vi "Read Array.vi"(8 "error in (no error)":errorcluster, 11 "JSON Value In":refnum<class "JSON Value.lvclass">) -> (0 "error out":errorcluster, 2 "Array":refnum<class "JSON Value.lvclass">[](array[class]), 3 "JSON Value Out":refnum<class "JSON Value.lvclass">)   [LabVIEW 2011, in "JSON Value.lvclass"]
doc: "Returns the elements of a JSON array as an array of <b>JSON Values</b>\n\nCopyright 2012 James David Powell, Shaun Rumbell and Ton Plomp\nMore information on http://lavag.org/topic/16217-cr-json-labview"
uses:
  JSON Value.lvclass
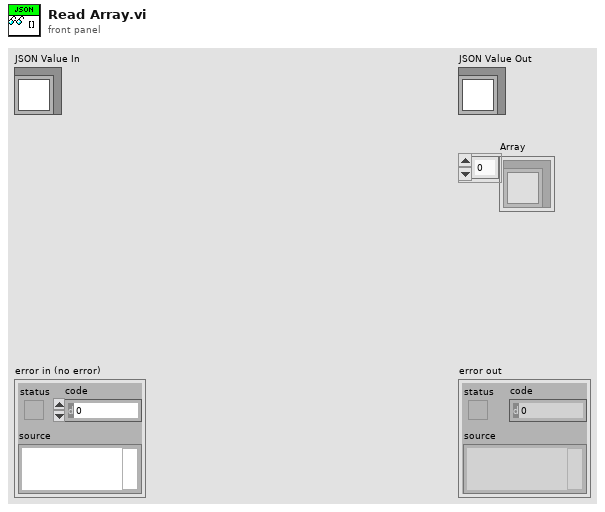
[diagram p1: front panel]
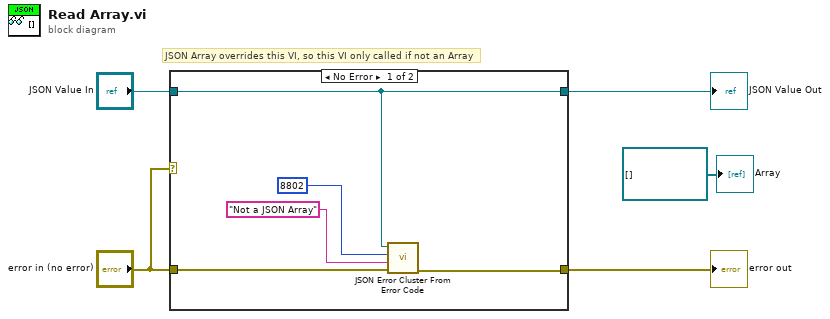
[diagram p0: block diagram]
diagram:
  # "JSON Array overrides this VI, so this VI only called if not an Array"
  n1 = case shown="No Error" "error in (no error)" {
    tunnel: "error in (no error)" -> [w8 w11]
    tunnel: [w7 w11] -> w5
    tunnel: "JSON Value In" -> [w6 w12]
    tunnel: [w6 w12] -> w3
    frame No Error {
      n2 = call "JSON Error Cluster From Error Code.vi"("error in (no error)"=w8, "Error message"="Not a JSON Array", "JSON error code"=8802, "JSON Value in"=w6) -> ("error out"=w7:errorcluster)  [unwired: 6 in, 1 out]
    }
    frame Error {
    }
  }
  "error out" <- w5
  "JSON Value Out" <- w3
  "Array" <- refnum<class "JSON Value.lvclass">[] [] ("Array")
